vi "ReadTxt_Tol_Table.vi"(4 "error in":errorcluster, 7 "ITmm path":path) -> (0 "error out":errorcluster, 1 "array_of_tolerances":dbl[][](array[numeric]))   [LabVIEW 2023]
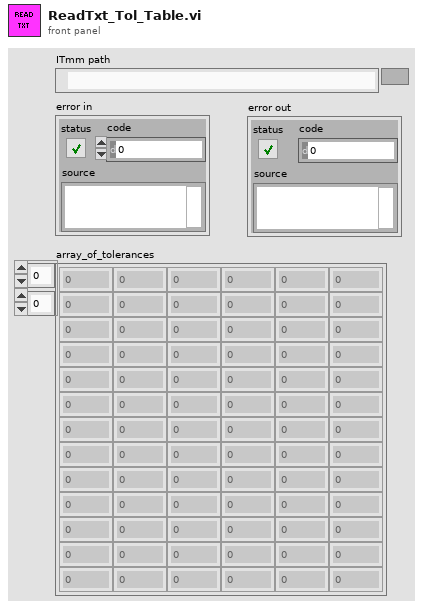
[diagram p1: front panel]
types:
  T1 = enum16{"open", "replace", "create", "open or create", "replace or create", "replace or create with confirmation"}
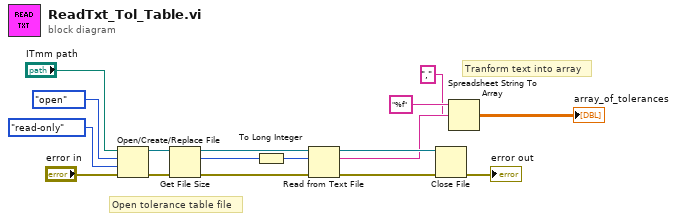
[diagram p0: block diagram]
diagram:
  # "Tranform text into array"
  # "Open tolerance table file"
  n1 = Open/Create/Replace File(file path (use dialog)="ITmm path", error in="error in", operation (0:open)=T1."open", access (0:read/write)=enum16{"read/write", "read-only", "write-only"}."read-only") -> (refnum out=w13:refnum<file>, error out=w14:errorcluster)  [unwired: 2 in, 1 out]
  n2 = Get File Size(file=w13, error in=w14) -> (refnum out=w9:refnum<file>, size (in bytes)=w12:i64, 0:w10:errorcluster)
  n3 = To Long Integer(number=w12) -> (32bit integer=w11:i32)
  n4 = Read from Text File(file (use dialog)=w9, count=w11, error in=w10) -> (refnum out=w8:refnum<file>, text=w4:string, error out=w7:errorcluster)  [unwired: 1 in, 1 out]
  n5 = Close File(refnum=w8, error in=w7) -> (error out=→"error out":errorcluster)  [unwired: 1 out]
  n6 = Spreadsheet String To Array(delimiter (Tab)=",", format string="%f", spreadsheet string=w4) -> (array=→"array_of_tolerances":dbl[][])  [unwired: 1 in]
